vi "OpenPowershell.vi"   [LabVIEW 2023, in "DeviceManager.lvclass"]
uses:
  DeviceManager.lvclass
  <vilib>/JKI/JKI DotNet System Exec/dotnet_system_exec/dotnet_system_exec.lvclass
panel:
  # "Locals"
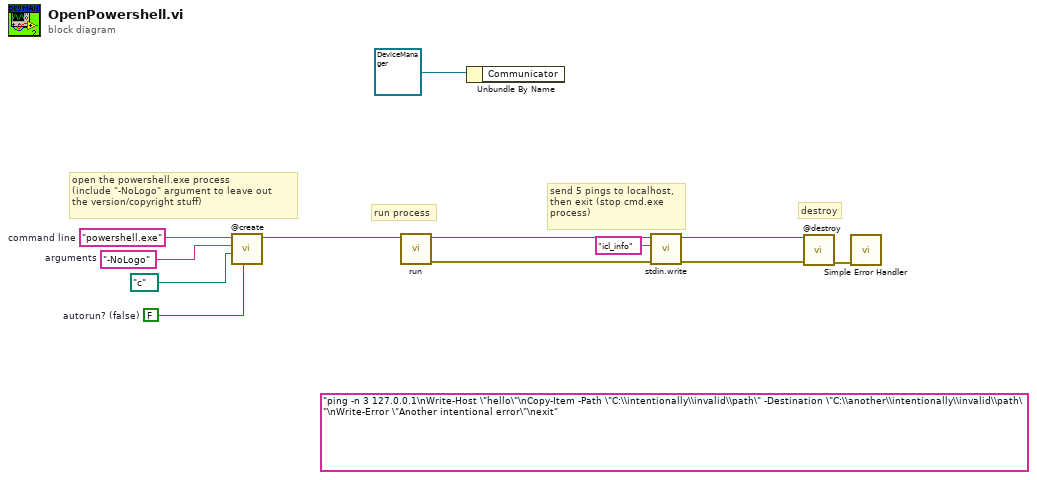
[diagram p0: block diagram]
diagram:
  (unwired) "ping -n 3 127.0.0.1\nWrite-Host \"hello\"\nCopy-Item -Path \"C:\\intentionally\\invalid\\path\" -Destination \"C:\\another\\intentionally\\invalid\\path\"\nWrite-Error \"Another intentional error\"\nexit" ("stdin")
  w8 = FALSE  # autorun? (false)
  w10 = "-NoLogo"  # arguments
  w11 = "powershell.exe"  # command line
  # "send 5 pings to localhost,\nthen exit (stop cmd.exe \nprocess)"
  # "destroy"
  # "run process"
  # "open the powershell.exe process\n(include \"-NoLogo\" argument to leave out\nthe version/copyright stuff)"
  n1 = call <vilib>:"@create.vi"("autorun? (false)"=w8, "working directory (c:\\)"=path "c:/" ("working directory"), "arguments (\"\")"=w10, "command line (cmd.exe)"=w11) -> ("dotnet_system_exec out"=w12:refnum<class "dotnet_system_exec.lvclass">)  [unwired: 5 in, 2 out]
  n2 = call <vilib>:"run.vi"("dotnet_system_exec in"=w12) -> ("error out"=w6:errorcluster, "dotnet_system_exec out"=w7:refnum<class "dotnet_system_exec.lvclass">)  [unwired: 9 in]
  n3 = Unbundle By Name(refnum<class "DeviceManager.lvclass"> refnum ("DeviceManager.lvclass")) -> ()  [unwired: 1 out]
  n4 = call-dynamic "stdin.write.vi"("error in (no error)"=w6, "stdin"="icl_info", "dotnet_system_exec in"=w7) -> ("error out"=w3:errorcluster, "dotnet_system_exec out"=w2:refnum<class "dotnet_system_exec.lvclass">)  [unwired: 7 in]
  n5 = call-dynamic "@destroy.vi"("error in (no error)"=w3, "dotnet_system_exec in"=w2) -> ("error out"=w4:errorcluster)  [unwired: 8 in, 1 out]
  n6 = call <vilib>:"Simple Error Handler.vi"("error in (no error)"=w4) -> ()  [unwired: 4 in, 5 out]
